vi "CSet_Control.vi"(8 "error in (no error)":errorcluster, 9 "CSet Control":T1(ring), 10 "CSet Filename (*.cal)":string, 11 "NetA_AgNA in":refnum<class "NetA_AgNA.lvclass">) -> (0 "error out":errorcluster, 2 "Current CSetName":string, 3 "NetA_AgNA out":refnum<class "NetA_AgNA.lvclass">)   [LabVIEW 2014, in "NetA_AgNA.lvclass"]
doc: "This allows user to load, save, or delete CalSet files. These files are proprietary and within the Keysight folders."
uses:
  NetA_AgNA.lvclass
  NetA_AgNA.lvclass/NetA_AgNA.ctl
  data/Agilent NA.lvlib
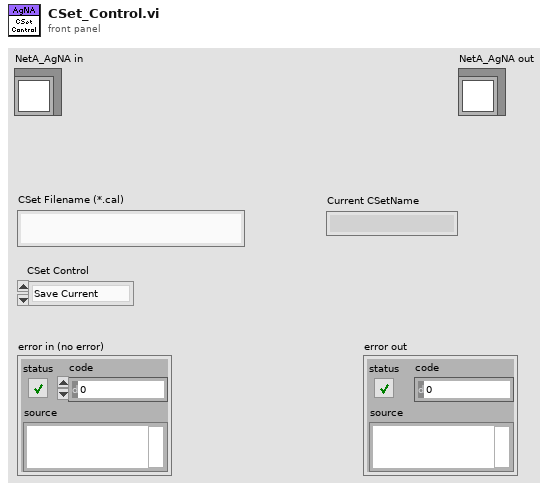
[diagram p1: front panel]
types:
  T1 = enum16{"Save Current", "Delete", "Apply", "Get Current"}
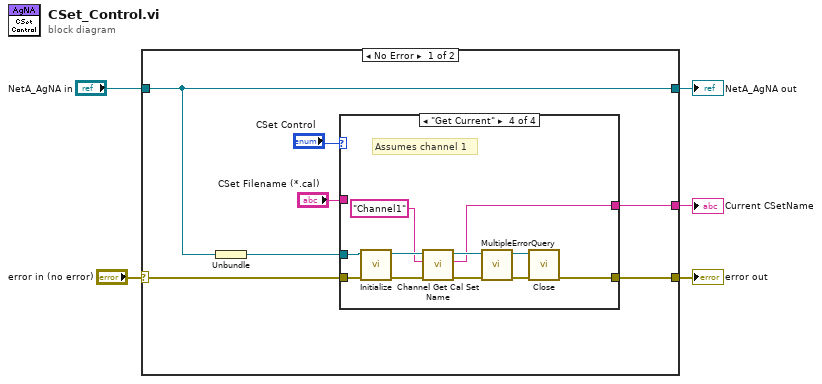
[diagram p0: block diagram]
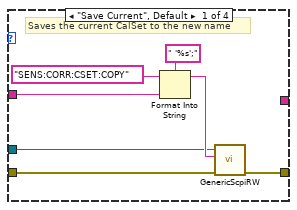
[diagram p2: hidden frame]
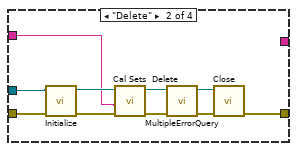
[diagram p3: hidden frame]
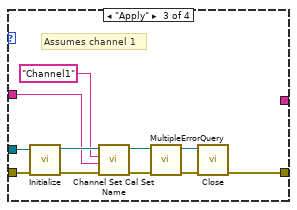
[diagram p4: hidden frame]
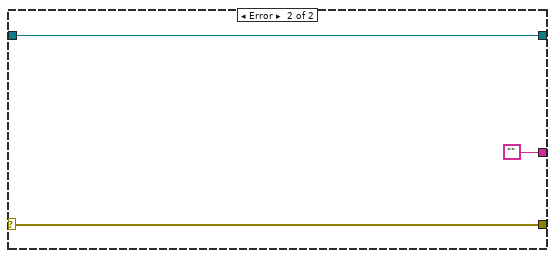
[diagram p5: hidden frame]
diagram:
  n1 = case shown="No Error" "error in (no error)" {
    selector: "error in (no error)" -> [w11 w53]
    tunnel: [w12 w53] -> w5
    tunnel: [w8 ""] -> w3
    tunnel: "NetA_AgNA in" -> [w7 w54]
    tunnel: [w7 w54] -> w1
    frame No Error {
      n2 = Unbundle(w7) -> (w6:refnum<k15>)
      n3 = case shown="\"Get Current\"" "CSet Control" {
        tunnel: [w19 w22 w37 w48] -> w12
        tunnel: w11 -> [w18 w29 w40 w51]
        tunnel: "CSet Filename (*.cal)" -> [w15 w21 w32 _]
        tunnel: [_ _ _ w42] -> w8
        tunnel: w6 -> [w13 w20 w30 w41]
        frame "Save Current", Default {
          # "Saves the current CalSet to the new name"
          n4 = Format Into String(format string=" '%s';", initial string="SENS:CORR:CSET:COPY" ("Get Dir List"), w15) -> (resulting string=w14:string)  [unwired: 1 in, 1 out]
          n5 = call "GenericScpiRW.vi"("error in (no error)"=w18, "SCPI Command"=w14, "resource name"=w13) -> ("error out"=w19:errorcluster)  [unwired: 7 in, 1 out]
        }
        frame "Delete" {
          n6 = call "Initialize.vi"("error in (no error)"=w29, "resource name"=w20) -> ("error out"=w25:errorcluster, "instrument handle out"=w28:refnum<k15>)  [unwired: 8 in]
          n7 = call "Cal Sets  Delete.vi"("error in (no error)"=w25, "CalSetName"=w21, "instrument handle"=w28) -> ("error out"=w24:errorcluster, "instrument handle out"=w27:refnum<k15>)  [unwired: 7 in]
          n8 = call "MultipleErrorQuery.vi"("error in (no error)"=w24, "instrument handle"=w27) -> ("error out"=w23:errorcluster, "instrument handle out"=w26:refnum<k15>)  [unwired: 7 in, 1 out]
          n9 = call "Close.vi"("error in (no error)"=w23, "instrument handle"=w26) -> ("error out"=w22:errorcluster)  [unwired: 9 in]
        }
        frame "Apply" {
          # "Assumes channel 1"
          n10 = call "Initialize.vi"("error in (no error)"=w40, "resource name"=w30) -> ("error out"=w36:errorcluster, "instrument handle out"=w35:refnum<k15>)  [unwired: 8 in]
          n11 = call "Channel Set Cal Set Name.vi"("error in (no error)"=w36, "CalSetName"=w32, "Channel"="Channel1", "instrument handle"=w35) -> ("error out"=w33:errorcluster, "instrument handle out"=w34:refnum<k15>)  [unwired: 6 in]
          n12 = call "MultipleErrorQuery.vi"("error in (no error)"=w33, "instrument handle"=w34) -> ("error out"=w38:errorcluster, "instrument handle out"=w39:refnum<k15>)  [unwired: 7 in, 1 out]
          n13 = call "Close.vi"("error in (no error)"=w38, "instrument handle"=w39) -> ("error out"=w37:errorcluster)  [unwired: 9 in]
        }
        frame "Get Current" {
          # "Assumes channel 1"
          n14 = call "Initialize.vi"("error in (no error)"=w51, "resource name"=w41) -> ("error out"=w47:errorcluster, "instrument handle out"=w44:refnum<k15>)  [unwired: 8 in]
          n15 = call "Channel Get Cal Set Name.vi"("error in (no error)"=w47, "Channel"="Channel1", "instrument handle"=w44) -> ("error out"=w46:errorcluster, "CalSetName"=w42:string, "instrument handle out"=w45:refnum<k15>)  [unwired: 6 in]
          n16 = call "MultipleErrorQuery.vi"("error in (no error)"=w46, "instrument handle"=w45) -> ("error out"=w49:errorcluster, "instrument handle out"=w50:refnum<k15>)  [unwired: 7 in, 1 out]
          n17 = call "Close.vi"("error in (no error)"=w49, "instrument handle"=w50) -> ("error out"=w48:errorcluster)  [unwired: 9 in]
        }
      }
    }
    frame Error {
    }
  }
  "error out" <- w5
  "Current CSetName" <- w3
  "NetA_AgNA out" <- w1
